vi "Tank Simulator.vi"(8 "error in (no error)":errorcluster, 10 "Flow Rate Data":string[][](array[string]), 11 "queue out":refnum<queue>) -> (0 "error in (no error) 2":errorcluster)   [LabVIEW 2024]
uses:
  Q Info.ctl
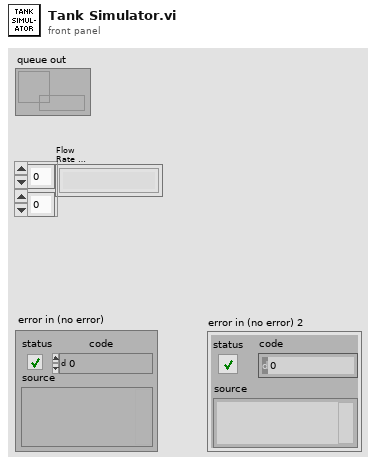
[diagram p1: front panel]
types:
  T1 = typedef "Q Info.ctl" = cluster{"State":string, "Data":variant}
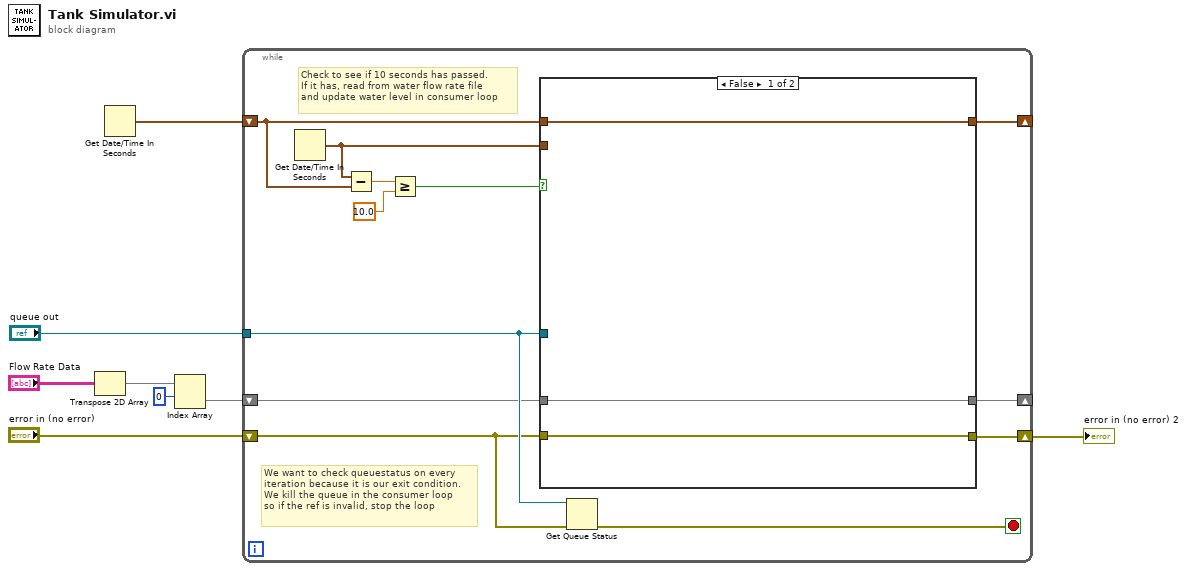
[diagram p0: block diagram]
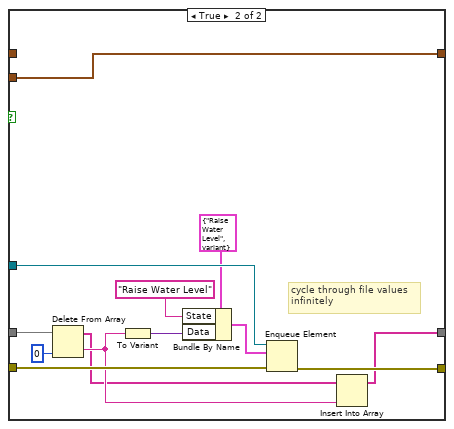
[diagram p2: hidden frame]
diagram:
  n1 = Transpose 2D Array(2D array="Flow Rate Data") -> (transposed array=w3:string[][])
  n2 = Get Date/Time In Seconds() -> (seconds since 1Jan1904=w6:timestamp)
  n3 = Index Array(array=w3, index (row)=0) -> (element=w1:string[])  [unwired: 1 in]
  n4 = while {
    tunnel: "queue out" -> [w16]
    shift-right: [w17] -> _
    shift-left: w6 -> [w11]
    shift-right: [w13] -> w7
    shift-left: "error in (no error)" -> [w14]
    shift-right: [w9] -> _
    shift-left: w1 -> [w10]
    stop <- w15 stop-if-true
    # "Check to see if 10 seconds has passed.\nIf it has, read from water flow rate file\nand update water level in consumer loop"
    # "We want to check queuestatus on every \niteration because it is our exit condition.\nWe kill the queue in the consumer loop\nso if the ref is invalid, stop the loop"
    n5 = Get Date/Time In Seconds() -> (seconds since 1Jan1904=w12:timestamp)
    n6 = Subtract(x=w12, y=w11) -> (x-y=w20:dbl)
    n7 = Greater Or Equal?(x=w20, y=10.0) -> (x >= y?=w18:bool)
    n8 = case shown="False" w18 {
      tunnel: w12 -> [_ w36]
      tunnel: [w23 w36] -> w17
      tunnel: w11 -> [w23 _]
      tunnel: w16 -> [_ w34]
      tunnel: w14 -> [w22 w35]
      tunnel: [w22 w29] -> w13
      tunnel: w10 -> [w21 w28]
      tunnel: [w21 w26] -> w9
      frame False {
      }
      frame True {
        # "cycle through file values\ninfinitely"
        n9 = Delete From Array(array=w28, index=0) -> (deleted portion=w27:string, array with subset deleted=w25:string[])  [unwired: 1 in]
        n10 = To Variant(anything=w27) -> (Variant=w32:variant)
        n11 = Bundle By Name(cluster=T1 {"State"="Raise Water Level", "Data"=variant} ("element"), "State"="Raise Water Level" ("String"), "Data"=w32) -> (w30:T1)
        n12 = Enqueue Element(queue=w34, element=w30, error in (no error)=w35) -> (error out=w29:errorcluster)  [unwired: 1 in, 2 out]
        n13 = Insert Into Array(array=w25, new element=w27) -> (w26:string[])  [unwired: 1 in]
      }
    }
    n14 = Get Queue Status(queue=w16, error in (no error)=w14) -> (error out=w15:errorcluster)  [unwired: 1 in, 7 out]
  }
  "error in (no error) 2" <- w7
